vi "histogram.vi"(1 "Steps":i32=13, 2 "intervals":i32=10, 3 "Data":dbl[][](array[numeric])) -> (0 "Array":cluster{"X Values":dbl[], dbl[]}[][](array[cluster]))   [LabVIEW 2021, in "CALIBRATION.lvlib"]
uses:
  CALIBRATION.lvlib
  <vilib>/Analysis/1siggen.llb/Ramp Pattern by Samples.vi
  <vilib>/gmath/statdist.llb/Normal PDF.vi
  <vilib>/Analysis/NI_AALBase.lvlib
  <vilib>/gmath/NI_Gmath.lvlib
panel:
  in  "index (row)":i32
  out "Histogram with PDF":cluster{"X Values":dbl[], dbl[]}[](graph)
  out "standard deviation":dbl format="%0.2f"
  out "mean":dbl format="%0.2f"
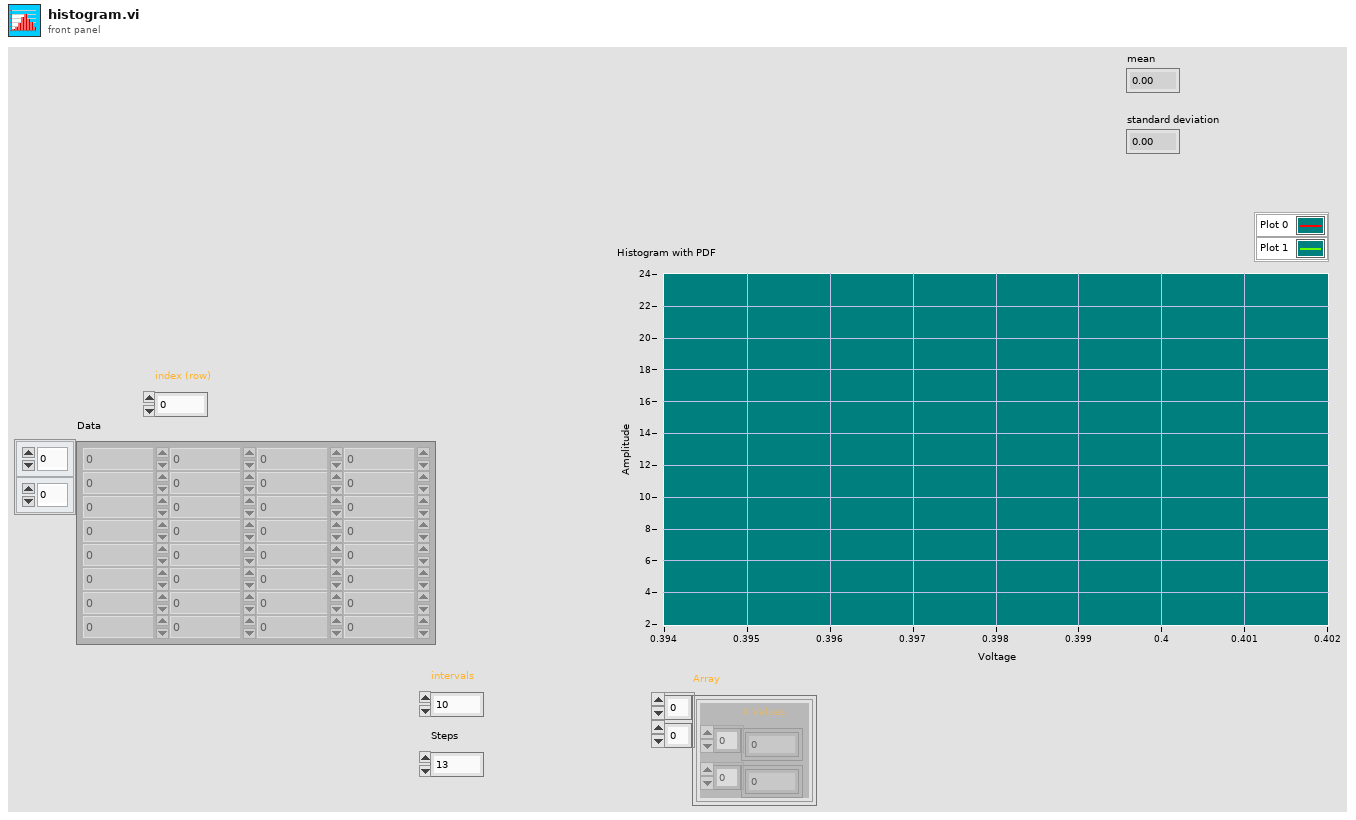
[diagram p1: front panel]
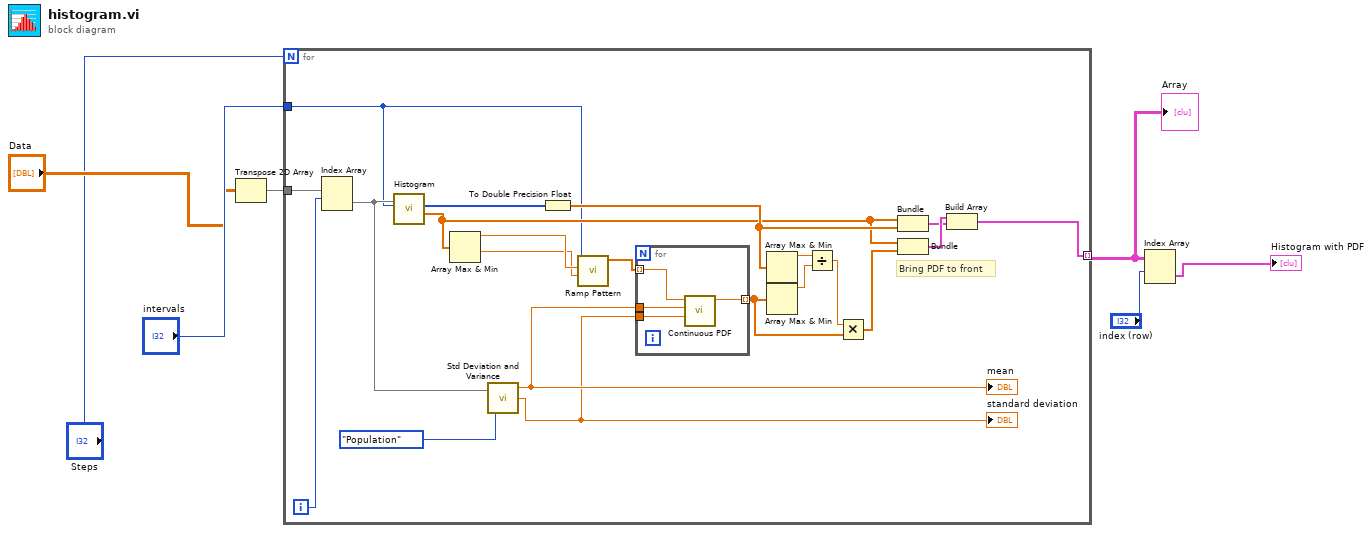
[diagram p0: block diagram]
diagram:
  n1 = Transpose 2D Array(2D array="Data") -> (transposed array=w7:dbl[][])
  n2 = for {
    N: "Steps" -> [_]
    tunnel: w7 -> [w16]
    tunnel: [w9] -> w6 mode=indexing
    tunnel: "intervals" -> [w8]
    i -> [w10]
    # "Bring PDF to front"
    n3 = Index Array(array=w16, index (row)=w10) -> (element=w15:dbl[])  [unwired: 1 in]
    n4 = call <vilib>:"Histogram.vi"("intervals"=w8, "X"=w15) -> ("X Values"=w11:dbl[], "Histogram: h(x)"=w25:i32[])  [unwired: 6 in, 2 out]
    n5 = Array Max & Min(array=w11) -> (max value=w14:dbl, min value=w13:dbl)  [unwired: 2 out]
    n6 = call <vilib>:"Std Deviation and Variance.vi"("X"=w15, "Weighting (Sample)"=enum16{"Sample", "Population"}."Population") -> ("mean"=w27:dbl, "standard deviation"=w26:dbl)  [unwired: 1 out]
    "mean" <- w27
    "standard deviation" <- w26
    n7 = To Double Precision Float(number=w25) -> (double precision float=w24:dbl[])
    n8 = call-poly <vilib>:"Ramp Pattern.vi"("start"=w13, "end"=w14, "samples"=w8) -> ("Ramp Pattern"=w12:dbl[])  [unwired: 7 in, 1 out]
    n9 = for {
      tunnel: w27 -> [w32]
      tunnel: w26 -> [w31]
      tunnel: [w30] -> w21 mode=indexing
      tunnel: w12 -> [w29] mode=indexing
      n10 = call-poly <vilib>:"Continuous PDF.vi"("std"=w31, "mean"=w32, "x"=w29) -> ("pdf(x)"=w30:dbl)  [unwired: 7 in, 1 out]
    }
    n11 = Array Max & Min(array=w24) -> (max value=w23:dbl)  [unwired: 3 out]
    n12 = Array Max & Min(array=w21) -> (max value=w22:dbl)  [unwired: 3 out]
    n13 = Divide(x=w23, y=w22) -> (x/y=w19:dbl)
    n14 = Multiply(x=w19, y=w21) -> (x*y=w20:dbl[])
    n15 = Bundle("X Values"=w11, w24) -> (w17:cluster{"X Values":dbl[], dbl[]})  [unwired: 1 in]
    n16 = Bundle("X Values"=w11, w20) -> (w18:cluster{"X Values":dbl[], dbl[]})  [unwired: 1 in]
    n17 = Build Array(w18, w17) -> (w9:cluster{"X Values":dbl[], dbl[]}[])
  }
  "Array" <- w6
  n18 = Index Array(array=w6, index (row)="index (row)") -> (element=→"Histogram with PDF":cluster{"X Values":dbl[], dbl[]}[])  [unwired: 1 in]
